vi "Read Data.vi"(6 "Port":T1, 7 "IP":i16, 8 "error in (no error)":errorcluster, 9 "Output":refnum<k21>, 10 "Instructions":refnum<k21>, 11 "MPU in":refnum<class "MPU.lvclass">) -> (0 "error out":errorcluster, 2 "IP Out":i16, 3 "MPU out":refnum<class "MPU.lvclass">)   [LabVIEW 2018, in "Modbus_Processing_Unit.lvlib" / "MPU.lvclass"]
uses:
  MPU.lvclass
  PortType.ctl
  MPU.lvclass/MPU.ctl
  <vilib>/rvi/DataTransferAndStorage/Container/Common/niFpgaContainerExecOnDevCompGetState.vi
  <vilib>/rvi/Emulation/niFpgaEmulationIsFPGAContextNoSignature.vi
  <vilib>/rvi/DataTransferAndStorage/Container/Common/niFpgaContainerGetUniqueNameForEmu.vi
  <vilib>/rvi/Emulation/niFpgaProcessEmulError.vi
  <vilib>/rvi/Emulation/niFpgaSctlEmulationGetInTimedLoop.vi
  <vilib>/rvi/errors/nirviReportUnexpectedCaseInternalError (U32).vi
  <vilib>/rvi/Memory/Memory_Emulation/niFpgaMemoryEmulationCacheClearOnFirstRun.vi
  <vilib>/rvi/Memory/Memory_Emulation/nirvimemoryEmulationManagerCache_MakeExclusive.vi
  <vilib>/rvi/Memory/Memory_Emulation/niFpgaMemoryEmulationValidateCache.vi
  <vilib>/rvi/Memory/Memory_Emulation/nirvimemoryEmulationManagerCache_InsertValue.vi
  <vilib>/Utility/error.llb/Clear Errors.vi
  <vilib>/rvi/Memory/Memory_Emulation/nirvimemoryEmulationManagerCache_ReleaseExclusive.vi
  <vilib>/rvi/Memory/Memory_Emulation/nirvimemoryEmulationManagerCache_GetValue.vi
  <vilib>/rvi/Memory/Memory_Emulation/nirvimemoryEmulationManagerCache_SetValue.vi
  <vilib>/rvi/Emulation/niFpgaSctlEmulationResourceMgr.vi
  <vilib>/rvi/Emulation/niFpgaGetClockAttributes.vi
  <vilib>/rvi/Emulation/niFpgaEmulationReportErrorSimple.vi
  <vilib>/rvi/Emulation/niFpgaCriticalErrorInLSC.vi
  <vilib>/rvi/DataTransferAndStorage/Container/XNode/niFpgaContainer.xnode
  <vilib>/rvi/Memory/Memory_Emulation/niFpgaMemoryEmulationRefIn.vi
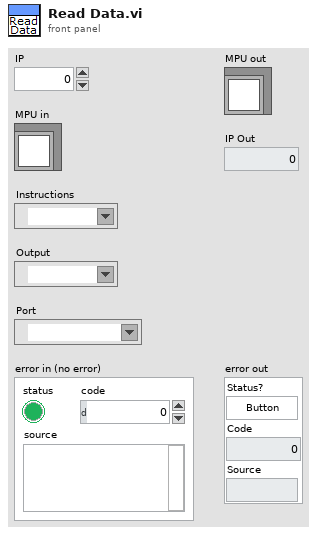
[diagram p1: front panel]
types:
  T1 = typedef "PortType.ctl" = refnum<k21>
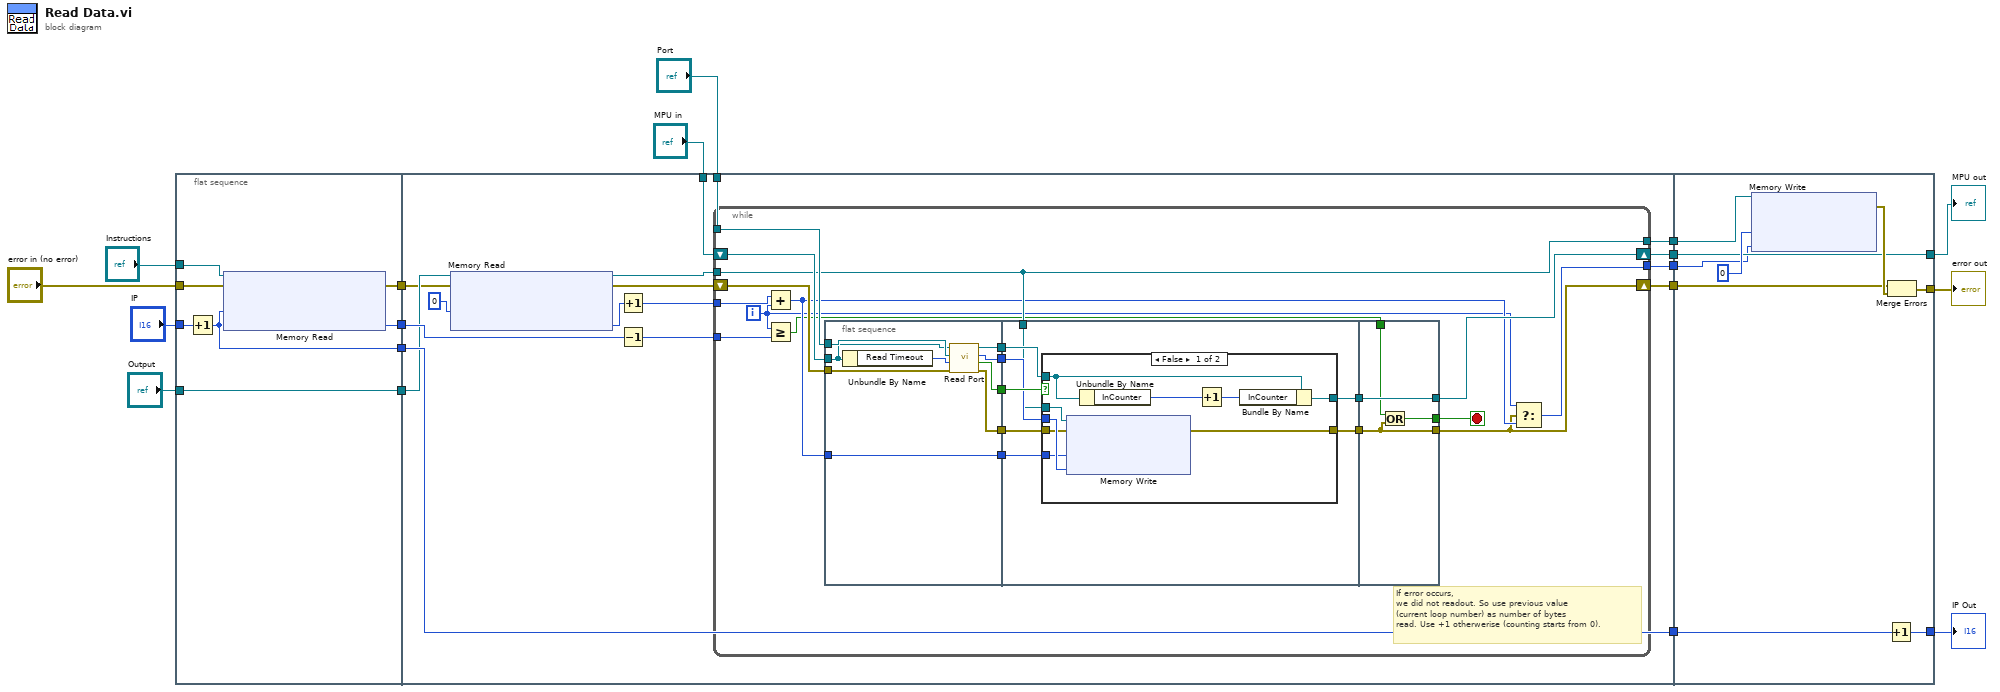
[diagram p0: block diagram]
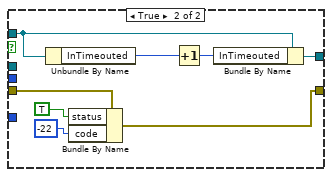
[diagram p2: hidden frame]
diagram:
  n1 = flat-sequence {
    tunnel: [w19] -> w18
    tunnel: "error in (no error)" -> [w22]
    tunnel: [w21] -> w17
    tunnel: "IP" -> [w25]
    tunnel: [w20] -> w16
    tunnel: "Output" -> [w24]
    tunnel: [w24] -> w15
    tunnel: "Instructions" -> [w23]
    tunnel: [w41] -> w14
    tunnel: w18 -> [w40]
    tunnel: w17 -> [w31]
    tunnel: w16 -> [w41]
    tunnel: w15 -> [w36]
    tunnel: "MPU in" -> [w39]
    tunnel: "Port" -> [w38]
    tunnel: [w33] -> w13
    tunnel: [w37] -> w12
    tunnel: [w35] -> w2
    tunnel: [w34] -> w1
    tunnel: [w101] -> w8
    tunnel: [w107] -> w4
    tunnel: w14 -> [w108]
    tunnel: w13 -> [w100]
    tunnel: w12 -> [w105]
    tunnel: [w103] -> w3
    tunnel: w2 -> [w103]
    tunnel: w1 -> [w102]
    frame #0 {
      n2 = Increment(x=w25) -> (x+1=w20:i16)
      n3 = xnode ("Memory Read")("Address"=w20, "error in (no error)"=w22, "Memory In"=w23) -> ("Data"=w19:u8, "error out"=w21:errorcluster)  [unwired: 1 out]
    }
    frame #1 {
      n4 = xnode "Memory Read"("Address"=u32 0, "error in (no error)"=w31, "Memory In"=w36) -> ("Data"=w28:u8, "error out"=w30:errorcluster, "Memory Out"=w32:refnum<k21>)
      n5 = Increment(x=w28) -> (x+1=w27:u8)
      n6 = Decrement(x=w40) -> (x-1=w26:u8)
      n7 = while {
        tunnel: w26 -> [w52]
        tunnel: w38 -> [w59]
        tunnel: w32 -> [w51]
        tunnel: [w51] -> w37
        shift-right: [w54] -> w35
        shift-left: w39 -> [w60]
        tunnel: [w50] -> w34
        shift-right: [w48] -> w33
        shift-left: w30 -> [w61]
        tunnel: w27 -> [w47]
        i -> [w46]
        stop <- w42 stop-if-true
        # "If error occurs,\nwe did not readout. So use previous value\n(current loop number) as number of bytes\nread. Use +1 otherwerise (counting starts from 0)."
        n8 = Add(x=w47, y=w46) -> (x+y=w49:i32)
        n9 = Greater Or Equal?(x=w46, y=w52) -> (x >= y?=w43:bool)
        n10 = flat-sequence {
          tunnel: w49 -> [w64]
          tunnel: w61 -> [w70]
          tunnel: w60 -> [w63]
          tunnel: w59 -> [w68]
          tunnel: [w69] -> w58
          tunnel: [w67] -> w57
          tunnel: [w66] -> w56
          tunnel: [w65] -> w55
          tunnel: [w64] -> w53
          tunnel: w58 -> [w78]
          tunnel: w57 -> [w77]
          tunnel: w56 -> [w75]
          tunnel: w55 -> [w74]
          tunnel: w51 -> [w73]
          tunnel: w53 -> [w71]
          tunnel: [w76] -> w45
          tunnel: [w72] -> w44
          tunnel: [w98] -> w48
          tunnel: [w99] -> w54
          tunnel: w45 -> [w99]
          tunnel: w44 -> [w98]
          tunnel: w43 -> [w97]
          tunnel: [w96] -> w42
          frame #0 {
            n11 = Unbundle By Name(w63) -> ("Read Timeout"=w62:u16)
            n12 = call-dynamic "Read Port.vi"("error in (no error)"=w70, "Timeout"=w62, "Port"=w68, "MPU in"=w63) -> ("error out"=w65:errorcluster, "Timeouted"=w67:bool, "Data"=w66:u8, "MPU out"=w69:refnum<class "MPU.lvclass">)  [unwired: 4 in]
          }
          frame #1 {
            n13 = case shown="False" w77 {
              tunnel: w78 -> [w80 w91]
              tunnel: [w81 w92] -> w76
              tunnel: w75 -> [w85 _]
              tunnel: w74 -> [w84 w93]
              tunnel: w73 -> [w83 _]
              tunnel: [w82 w90] -> w72
              tunnel: w71 -> [w79 _]
              frame False {
                n14 = xnode ("Memory Write")("error in (no error)"=w84, "Memory In"=w83, "Address"=w79, "Data"=w85) -> ("error out"=w82:errorcluster)  [unwired: 1 out]
                n15 = Unbundle By Name(w80) -> ("InCounter"=w87:u64)
                n16 = Increment(x=w87) -> (x+1=w86:u64)
                n17 = Bundle By Name(cluster=w80, "InCounter"=w86) -> (w81:refnum<class "MPU.lvclass">)
              }
              frame True {
                n18 = Unbundle By Name(w91) -> ("InTimeouted"=w95:u64)
                n19 = Bundle By Name(cluster=w93, "status"=TRUE, "code"=-22) -> (w90:errorcluster)
                n20 = Increment(x=w95) -> (x+1=w94:u64)
                n21 = Bundle By Name(cluster=w91, "InTimeouted"=w94) -> (w92:refnum<class "MPU.lvclass">)
              }
            }
          }
          frame #2 {
            n22 = Or(x=w97, y=w98) -> (x .or. y?=w96:bool)
          }
        }
        n23 = Select(t=w46, s=w48, f=w49) -> (s? t:f=w50:i32)
      }
    }
    frame #2 {
      n24 = xnode ("Memory Write")("Address"=u32 0, "Data"=w102, "Memory In"=w105) -> ("error out"=w106:errorcluster)  [unwired: 1 in, 1 out]
      n25 = Increment(x=w108) -> (x+1=w107:i16)
      n26 = Merge Errors(w100, w106) -> (w101:errorcluster)
    }
  }
  "MPU out" <- w3
  "error out" <- w8
  "IP Out" <- w4
